vi "Configure Multi-Point [MP].vi"(5 "sample interval (0.0 s)":dbl format="%.3f", 7 "sample trigger (Immediate)":i32(ring)=1 items=["Immediate"=1, "External"=2, "Software Trigger Function"=3, "Interval"=10, "PXI TRIG0 or VXI TTL0"=111, "PXI TRIG1 or VXI TTL1"=112, "PXI TRIG2 or VXI TTL2"=113, "PXI TRIG3 or VXI TTL3"=114, "PXI TRIG4 or VXI TTL4"=115, "PXI TRIG5 or VXI TTL5"=116, "PXI TRIG6 or VXI TTL6"=117, "PXI TRIG7 or VXI TTL7"=118, "ECL0"=119, "ECL1"=120, "PXI Star"=131, "RTSI 0"=140, "RTSI 1"=141, "RTSI 2"=142, "RTSI 3"=143, "RTSI 4"=144, "RTSI 5"=145, "RTSI 6"=146], 8 "error in (no error)":errorcluster, 9 "sample count (1)":i32=1, 10 "trigger count (1)":i32=1, 11 "CS++DMM in":refnum<class "CS++DMM.lvclass">) -> (0 "error out":errorcluster, 3 "CS++DMM out":refnum<class "CS++DMM.lvclass">)   [LabVIEW 2013, in "CS++DMM.lvlib" / "CS++DMM.lvclass"]
doc: "This VI configures the properties that affect multi-point measurements. These properties are the trigger count, sample count, sample trigger and sample interval.\n\nNote:\n\n(1) This VI is part of the IviDmmMultiPoint [MP] extension group."
uses:
  CS++DMM.lvclass
  Core/Classes/CS++ProcessVariables/ProcessVariable/PV.lvclass
  CS++DMM.lvclass/CS++DMM.ctl
  Core/Classes/CS++ProcessVariables/PVConnection/PVConnection.lvclass
  Core/Classes/CS++ProcessVariables/ProcessVariable/PV.lvclass/PV.ctl
  Core/Classes/CS++ProcessVariables/ProcessVariable/Write Data.vi
  Core/Classes/CS++ProcessVariables/ProcessVariable/Write Timestamp.vi
  Core/Classes/CS++ProcessVariables/ProcessVariable/Write Quality.vi
  Core/Classes/CS++ProcessVariables/ProcessVariable/Write status.vi
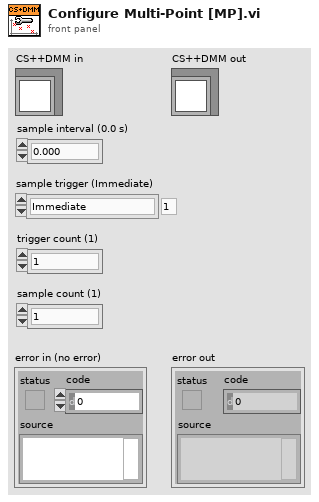
[diagram p1: front panel]
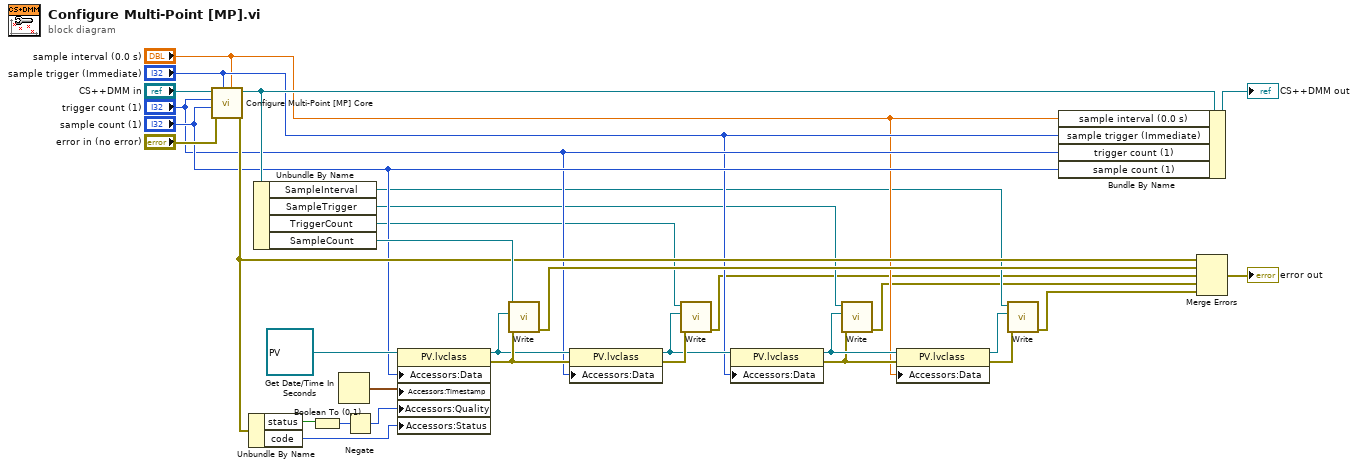
[diagram p0: block diagram]
diagram:
  n1 = call-dynamic "Configure Multi-Point [MP] Core.vi"("sample interval (0.0 s)"="sample interval (0.0 s)", "sample trigger (Immediate)"="sample trigger (Immediate)", "error in (no error)"="error in (no error)", "sample count (1)"="sample count (1)", "trigger count (1)"="trigger count (1)", "CS++DMM in"="CS++DMM in") -> ("error out"=w21:errorcluster, "CS++DMM out"=w20:refnum<class "CS++DMM.lvclass">)  [unwired: 4 in]
  n2 = Unbundle By Name(w21) -> ("status"=w30:bool, "code"=w27:i32)
  n3 = Unbundle By Name(w20) -> ("SampleInterval"=w4:refnum<class "PVConnection.lvclass">, "SampleTrigger"=w10:refnum<class "PVConnection.lvclass">, "TriggerCount"=w13:refnum<class "PVConnection.lvclass">, "SampleCount"=w32:refnum<class "PVConnection.lvclass">)
  n4 = Boolean To (0,1)(Boolean=w30) -> (0, 1=w29:i16)
  n5 = Get Date/Time In Seconds() -> (seconds since 1Jan1904=w26:timestamp)
  n6 = Negate(x=w29) -> (-x=w28:i16)
  n7 = property class="PV.lvclass"(reference=refnum<class "PV.lvclass"> refnum ("CS++ProcessVariables.lvlib:PV.lvclass"), "Accessors:Data"="sample count (1)", "Accessors:Timestamp"=w26, "Accessors:Quality"=w28, "Accessors:Status"=w27) -> (reference out=w15:refnum<class "PV.lvclass">, error out=w16:errorcluster)  [unwired: 1 in]
  n8 = call-dynamic "Write.vi"("error in (no error)"=w16, "PV"=w15, "PVConnection in"=w32) -> ("error out"=w25:errorcluster)  [unwired: 7 in, 1 out]
  n9 = property class="PV.lvclass"(reference=w15, error in=w16, "Accessors:Data"="trigger count (1)") -> (reference out=w12:refnum<class "PV.lvclass">, error out=w17:errorcluster)
  n10 = call-dynamic "Write.vi"("error in (no error)"=w17, "PV"=w12, "PVConnection in"=w13) -> ("error out"=w3:errorcluster)  [unwired: 7 in, 1 out]
  n11 = property class="PV.lvclass"(reference=w12, "Accessors:Data"="sample trigger (Immediate)") -> (reference out=w7:refnum<class "PV.lvclass">, error out=w6:errorcluster)  [unwired: 1 in]
  n12 = call-dynamic "Write.vi"("error in (no error)"=w6, "PV"=w7, "PVConnection in"=w10) -> ("error out"=w2:errorcluster)  [unwired: 7 in, 1 out]
  n13 = property class="PV.lvclass"(reference=w7, error in=w6, "Accessors:Data"="sample interval (0.0 s)") -> (reference out=w8:refnum<class "PV.lvclass">, error out=w9:errorcluster)
  n14 = call-dynamic "Write.vi"("error in (no error)"=w9, "PV"=w8, "PVConnection in"=w4) -> ("error out"=w1:errorcluster)  [unwired: 7 in, 1 out]
  n15 = Bundle By Name(cluster=w20, "sample interval (0.0 s)"="sample interval (0.0 s)", "sample trigger (Immediate)"="sample trigger (Immediate)", "trigger count (1)"="trigger count (1)", "sample count (1)"="sample count (1)") -> (→"CS++DMM out":refnum<class "CS++DMM.lvclass">)
  n16 = Merge Errors(w21, w25, w3, w2, w1) -> (→"error out":errorcluster)
